vi "Delete Panel.vi"(8 "error in":errorcluster caption="错误输入（无错误）", 9 "Abort VI":bool, 10 "SelfNode*":refnum<data-value>) -> (0 "error out":errorcluster caption="错误输出", 2 "BrotherNodeBeDeleted":refnum<data-value>, 3 "ParentNode*":refnum<data-value>)   [LabVIEW 2016, in "PanelDataNode.lvclass"]
uses:
  PanelDataNode.lvclass
  C:/Users/CL/Desktop/ZcDAQprj0811/ZcDAQprj/Modules/DAQ-Display/PanelSplitToolkit/PanelLinkNode/PanelLinkNode.lvclass
  PanelObject/PanelObject.lvclass
  PanelLinkNode/PanelLinkNode.lvclass/PanelLinkNode.ctl
  PanelLinkNode/PanelLinkNode.lvclass
  C:/Users/CL/Desktop/ZcDAQprj0811/ZcDAQprj/Modules/DAQ-Display/PanelSplitToolkit/PanelObject/PanelObject.lvclass
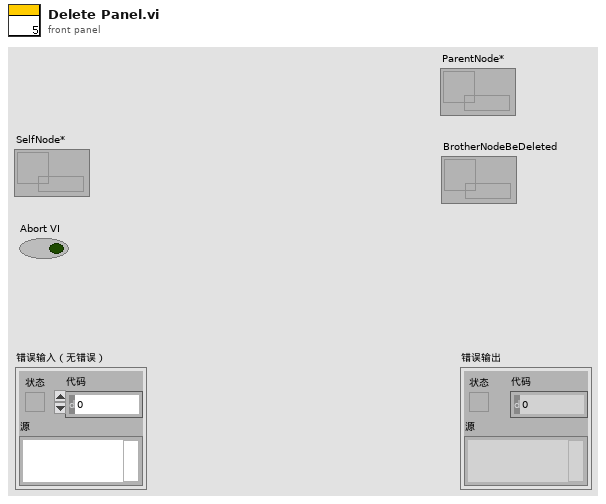
[diagram p1: front panel]
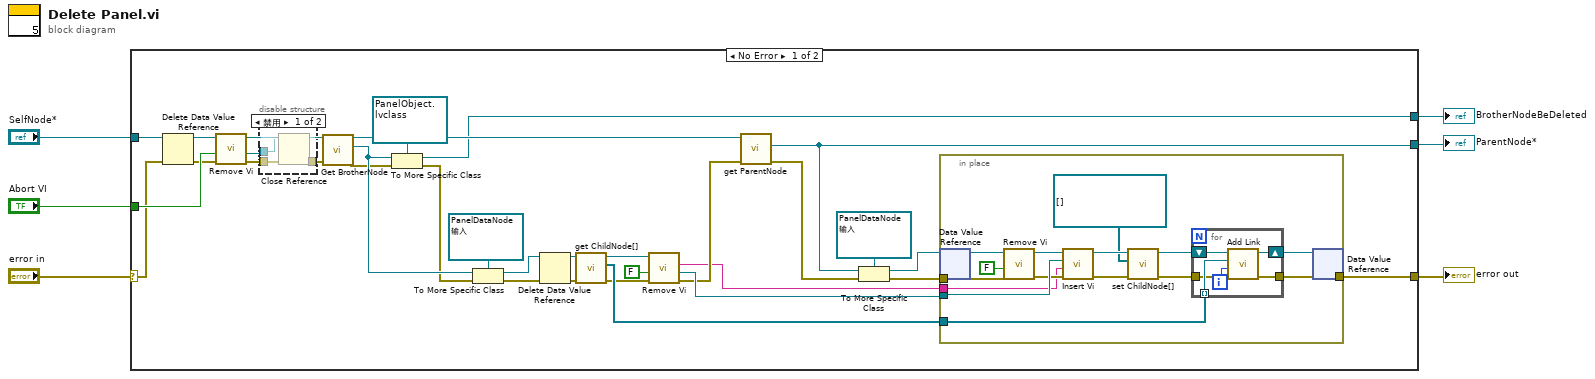
[diagram p0: block diagram]
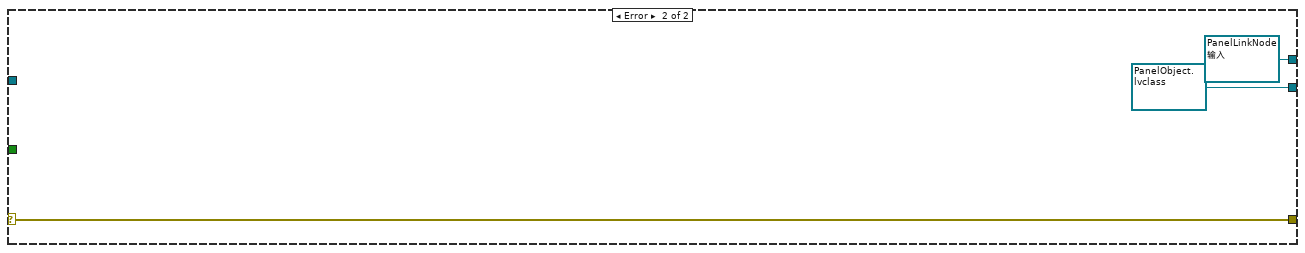
[diagram p3: hidden frame]
diagram:
  n1 = case shown="No Error" "error in" {
    selector: "error in" -> [w7 w67]
    tunnel: [w39 w67] -> w5
    tunnel: "SelfNode*" -> [w19 _]
    tunnel: "Abort VI" -> [w38 _]
    tunnel: [w12 refnum<data-value> refnum ("BrotherNode*")] -> w2
    tunnel: [w10 refnum<data-value> refnum ("ParentNode*")] -> w1
    frame No Error {
      n2 = Delete Data Value Reference(data value reference=w19, error in=w7) -> (data value=w18:refnum<class "PanelDataNode.lvclass">, error out=w17:errorcluster)
      n3 = call-dynamic "Remove Vi.vi"("error in"=w17, "Abort VI"=w38, "PanelDataNode 输入"=w18) -> ("error out"=w31:errorcluster, "VI*"=w14:refnum<vi>, "PanelDataNode 输出"=w35:refnum<class "PanelDataNode.lvclass">)  [unwired: 5 in, 1 out]
      n4 = disable-structure shown="禁用" {
        disable-tunnel: w31 -> [w42 w43]
        disable-tunnel: [w41 w43] -> w15
        disable-tunnel: w14 -> [w40 _]
        frame Disabled {
          n5 = Close Reference(reference=w40, error in (no error)=w42) -> (error out=w41:errorcluster)
        }
        frame Enabled {
        }
      }
      n6 = call-dynamic "Get BrotherNode.vi"("error in (no error)"=w15, "PanelLinkNode 输入"=w35) -> ("error out"=w9:errorcluster, "BrotherNode*"=w13:refnum<data-value>, "PanelLinkNode 输出"=w33:refnum<class "PanelDataNode.lvclass">)  [unwired: 7 in]
      n7 = To More Specific Class(target class=refnum<data-value> refnum ("ChildNode*"), reference=w13, error in=w9) -> (specific class reference=w12:refnum<data-value>, error out=w8:errorcluster)
      n8 = To More Specific Class(target class=refnum<data-value> refnum ("SelfNode*"), reference=w13, error in=w8) -> (specific class reference=w24:refnum<data-value>, error out=w22:errorcluster)
      n9 = Delete Data Value Reference(data value reference=w24, error in=w22) -> (data value=w23:refnum<class "PanelDataNode.lvclass">, error out=w21:errorcluster)
      n10 = call "get ChildNode[].vi"("error in (no error)"=w21, "PanelLinkNode输入"=w23) -> ("error out"=w26:errorcluster, "ChildNode*[]"=w28:refnum<data-value>[], "PanelLinkNode输出"=w27:refnum<class "PanelDataNode.lvclass">)  [unwired: 7 in]
      n11 = call-dynamic "Remove Vi.vi"("error in"=w26, "Abort VI"=FALSE, "PanelDataNode 输入"=w27) -> ("error out"=w20:errorcluster, "VI*"=w32:refnum<vi>, "ViValue"=w16:string)  [unwired: 5 in, 1 out]
      n12 = call "get ParentNode.vi"("error in (no error)"=w20, "PanelLinkNode输入"=w33) -> ("error out"=w30:errorcluster, "ParentNode*"=w10:refnum<data-value>)  [unwired: 7 in, 1 out]
      n13 = To More Specific Class(target class=refnum<data-value> refnum ("SelfNode*"), reference=w10, error in=w30) -> (specific class reference=w36:refnum<data-value>, error out=w29:errorcluster)
      n14 = in-place {
        in-place-border: w32 -> [w56]
        in-place-border: w29 -> [w54]
        in-place-border: [w50] -> w39
        in-place-border: w28 -> [w51]
        in-place-border: w16 -> [w44]
        n15 = in-place-dvr #1(w36) -> (w58:refnum<class "PanelDataNode.lvclass">)  [unwired: 1 out]
        n16 = call-dynamic "Remove Vi.vi"("error in"=w54, "Abort VI"=FALSE, "PanelDataNode 输入"=w58) -> ("error out"=w55:errorcluster, "PanelDataNode 输出"=w57:refnum<class "PanelDataNode.lvclass">)  [unwired: 5 in, 2 out]
        n17 = call-dynamic "Insert Vi.vi"("error in (no error)"=w55, "ViValue"=w44, "VI*"=w56, "PanelDataNode 输入"=w57) -> ("error out"=w47:errorcluster, "PanelDataNode 输出"=w49:refnum<class "PanelDataNode.lvclass">)  [unwired: 6 in]
        n18 = call "set ChildNode[].vi"("error in (no error)"=w47, "ChildNode*[]"=refnum<data-value>[] [], "PanelLinkNode输入"=w49) -> ("error out"=w46:errorcluster, "PanelLinkNode输出"=w48:refnum<class "PanelDataNode.lvclass">)  [unwired: 7 in]
        n19 = for {
          tunnel: w51 -> [w62] mode=indexing
          tunnel: w46 -> [w61]
          tunnel: [w60] -> w50
          shift-right: [w63] -> w52
          shift-left: w48 -> [w64]
          i -> [w59]
          n20 = call-dynamic "Add Link.vi"("ParentLinkNode in"=w64, "ChildNode* in"=w62, "L\\R Child"=w59, "error in (no error)"=w61) -> ("ParentLinkNode out"=w63:refnum<class "PanelDataNode.lvclass">, "error out"=w60:errorcluster)  [unwired: 5 in]
        }
        n21 = in-place-dvr #1(w52) -> ()  [unwired: 2 out]
      }
    }
    frame Error {
    }
  }
  "error out" <- w5
  "BrotherNodeBeDeleted" <- w2
  "ParentNode*" <- w1
